vi "Side Location.vi"(8 "error in (no error)":errorcluster, 10 "Enum":enum16{"MaxToStander", "StanderToMax"}(ring), 11 "UI_Top_Customer in":refnum<class "UI_Top_Customer.lvclass">) -> (0 "error out":errorcluster, 3 "UI_Top_Customer out":refnum<class "UI_Top_Customer.lvclass">)   [LabVIEW 2021, in "UI_Top_Customer.lvclass"]
uses:
  UI_Top_Customer.lvclass
  C:/Program Files (x86)/National Instruments/LabVIEW 2021/user.lib/John_Lib/AbstractActorTemplate/AbstractActorTemplate/UIActorTop.lvclass
  <vilib>/Utility/miscctls.llb/LVRectTypeDef.ctl
  <vilib>/Utility/miscctls.llb/LVBoundsTypeDef.ctl
  <vilib>/Utility/miscctls.llb/LVPositionTypeDef.ctl
  UI_Top_Customer.lvclass/UI_Top_Customer.ctl
panel:
  out "Array":T1[](array[typedef])
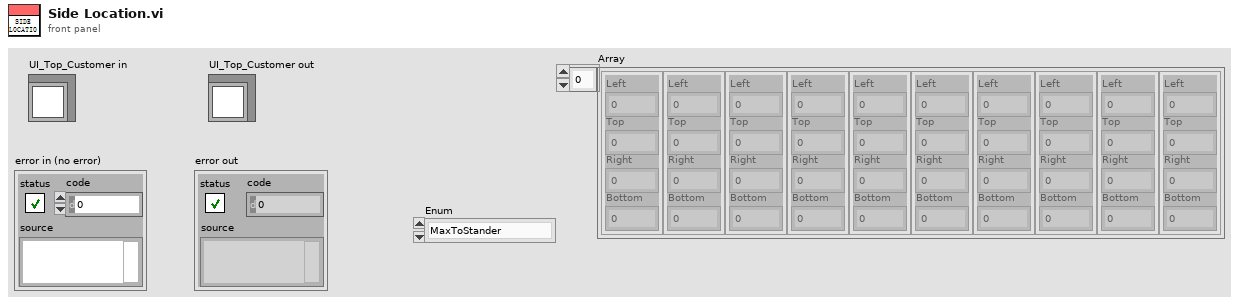
[diagram p1: front panel]
types:
  T1 = typedef "LVRectTypeDef.ctl" = cluster{"Left":i16, "Top":i16, "Right":i16, "Bottom":i16}
  T2 = typedef "LVPositionTypeDef.ctl" = cluster{"Left":i32, "Top":i32}
  T3 = typedef "LVBoundsTypeDef.ctl" = cluster{"Width":u32, "Height":u32}
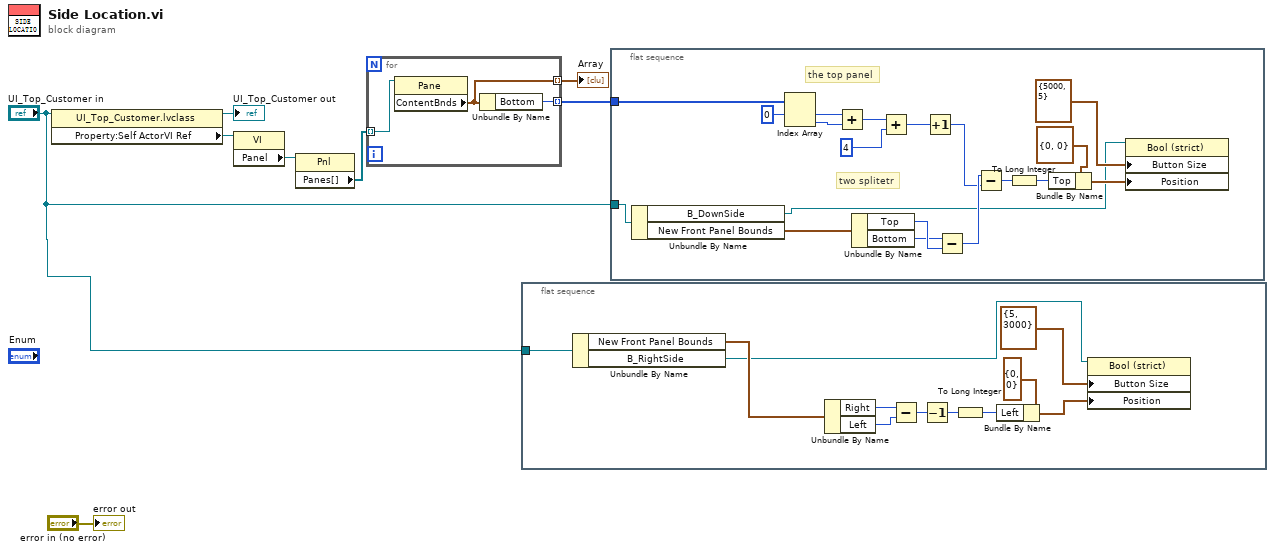
[diagram p0: block diagram]
diagram:
  n1 = property class="UI_Top_Customer.lvclass"(reference="UI_Top_Customer in") -> (reference out=→"UI_Top_Customer out":refnum<class "UI_Top_Customer.lvclass">, "Property:Self ActorVI Ref"=w5:refnum<vi>)  [unwired: 1 in, 1 out]
  n2 = property class="VI"(reference=w5) -> ("Panel"=w7:refnum<vi>)  [unwired: 1 in, 2 out]
  n3 = property class="Pnl"(reference=w7) -> ("Panes[]"=w4:refnum<vi>[])  [unwired: 1 in, 2 out]
  n4 = for {
    tunnel: w4 -> [w11] mode=indexing
    tunnel: [w10] -> w3 mode=indexing
    tunnel: [w9] -> w2 mode=indexing
    n5 = property class="Pane"(reference=w11) -> ("ContentBnds"=w10:T1)  [unwired: 1 in, 2 out]
    n6 = Unbundle By Name(w10) -> ("Bottom"=w9:i16)
  }
  "Array" <- w3
  n7 = flat-sequence {
    tunnel: "UI_Top_Customer in" -> [w14]
    frame #0 {
      n8 = Unbundle By Name(w14) -> ("New Front Panel Bounds"=w13:T1, "B_RightSide"=w12:refnum<vi>)
      n9 = Unbundle By Name(w13) -> ("Right"=w16:i16, "Left"=w15:i16)
      n10 = Subtract(x=w16, y=w15) -> (x-y=w19:i16)
      n11 = Decrement(x=w19) -> (x-1=w18:i16)
      n12 = To Long Integer(number=w18) -> (32bit integer=w17:i32)
      n13 = Bundle By Name(cluster=T2 {"Left"=0, "Top"=0} ("Position"), "Left"=w17) -> (w20:T2)
      n14 = property class="Bool (strict)"(reference=w12, "Button Size"=T3 {"Width"=5, "Height"=3000}, "Position"=w20) -> ()  [unwired: 1 in, 2 out]
    }
  }
  n15 = flat-sequence {
    tunnel: w2 -> [w34]
    tunnel: "UI_Top_Customer in" -> [w25]
    frame #0 {
      # "two splitetr"
      # "the top panel"
      n16 = Unbundle By Name(w25) -> ("B_DownSide"=w23:refnum<vi>, "New Front Panel Bounds"=w24:T1)
      n17 = Index Array(array=w34, index #1=0 ("index")) -> (element #1=w32:i16, element #2=w31:i16)  [unwired: 1 in]
      n18 = Add(x=w32, y=w31) -> (x+y=w30:i16)
      n19 = Unbundle By Name(w24) -> ("Top"=w37:i16, "Bottom"=w36:i16)
      n20 = Add(x=w30, y=i16 4) -> (x+y=w28:i16)
      n21 = Increment(x=w28) -> (x+1=w27:i16)
      n22 = Subtract(x=w36, y=w37) -> (x-y=w35:i16)
      n23 = Subtract(x=w35, y=w27) -> (x-y=w38:i16)
      n24 = To Long Integer(number=w38) -> (32bit integer=w26:i32)
      n25 = Bundle By Name(cluster=T2 {"Left"=0, "Top"=0} ("Position"), "Top"=w26) -> (w41:T2)
      n26 = property class="Bool (strict)"(reference=w23, "Button Size"=T3 {"Width"=5000, "Height"=5}, "Position"=w41) -> ()  [unwired: 1 in, 2 out]
    }
  }
  "error out" <- "error in (no error)"
